vi "Make Path Outcome Rectangles.vi"(5 "[user-specified font]":T2, 8 "Outcome Name":string, 9 "Path Name":string, 10 "Height Padding":dbl, 11 "Drawing Info":T3) -> (2 "Outcome Name Rect":T1, 3 "Path Name Rect":T1)   [LabVIEW 2025]
uses:
  <vilib>/Analysis/baseanly.llb/Mean (DBL).vi
  <vilib>/Analysis/NI_AALBase.lvlib
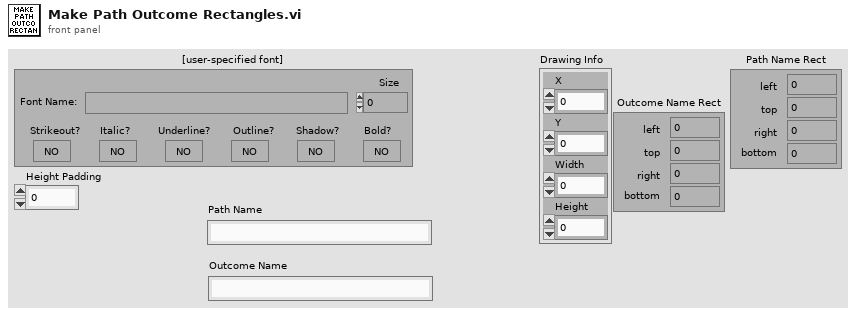
[diagram p1: front panel]
types:
  T1 = cluster{"left":i16, "top":i16, "right":i16, "bottom":i16}
  T2 = cluster{"Font Name:":string, "Size":i16, "Strikeout?":bool, "Italic?":bool, "Underline?":bool, "Outline?":bool, "Shadow?":bool, "Bold?":bool}
  T3 = cluster{"X":dbl, "Y":dbl, "Width":dbl, "Height":dbl}
  T4 = cluster{"horizontal":enum16{"left", "center", "right"}, "vertical":enum16{"top", "center", "bottom"}}
  T5 = enum16{"User-specified Font", "Application Font", "System Font", "Dialog Font"}
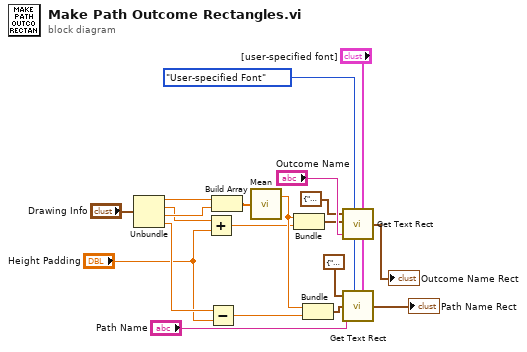
[diagram p0: block diagram]
diagram:
  w12 = T5."User-specified Font" ("desired font(Application)")
  n1 = Unbundle("Drawing Info") -> ("X"=w18:dbl, "Y"=w6:dbl, "Width"=w17:dbl, "Height"=w4:dbl)
  n2 = Add(x=w6, y="Height Padding") -> (x+y=w5:dbl)
  n3 = Subtract(x=w4, y="Height Padding") -> (x-y=w2:dbl)
  n4 = Build Array(w18, w17) -> (w16:dbl[])
  n5 = call-poly <vilib>:"Mean.vi"("X"=w16) -> ("mean"=w7:dbl)  [unwired: 1 out]
  n6 = Bundle("mean"=w7, w5) -> (w14:cluster{"mean":dbl, dbl})  [unwired: 1 in]
  n7 = Bundle("mean"=w7, w2) -> (w9:cluster{"mean":dbl, dbl})  [unwired: 1 in]
  n8 = call <vilib>:"Get Text Rect.vi"("alignment(left, top)"=T4 {"horizontal"=enum."center", "vertical"=enum."top"}, "desired font(Application)"=w12, "origin(0,0)"=w14, "text"="Outcome Name", "[user-specified font]"="[user-specified font]") -> ("rect"=→"Outcome Name Rect":T1)  [unwired: 4 in]
  n9 = call <vilib>:"Get Text Rect.vi"("alignment(left, top)"=T4 {"horizontal"=enum."center", "vertical"=enum."bottom"}, "desired font(Application)"=w12, "origin(0,0)"=w9, "text"="Path Name", "[user-specified font]"="[user-specified font]") -> ("rect"=→"Path Name Rect":T1)  [unwired: 4 in]
